vi "VoltageTest_R_VDC15V.vi"(0 "datain":string[](array[string])=["备注", "负载通道", "负载地址", "延时时间", "output max", "output min", "量测类型", "待测物板号"], 5 "HW CH Number":i32, 7 "Setup":string) -> (4 "REPORT INDECATE":string[][](array[string])=[["微安测试", "", "", "", ""], ["微安量测", "4", "0.000", "0.1", "NG"], ["微安量测", "4", "0.000", "0.1", "NG"], ["微安量测", "4", "0.000", "0.1", "NG"], ["微安量测", "4", "0.000", "0.1", "NG"]], 6 "ROW HEAD":string[](array[string]), 8 "PF":string[](array[string]), 10 "testData":string[](array[string]), 15 "Array":string[](array[string]))   [LabVIEW 2018]
uses:
  Subvi/Global.vi
panel:
  out "测试板数":i32
  out "数组":bool[](array[boolean])
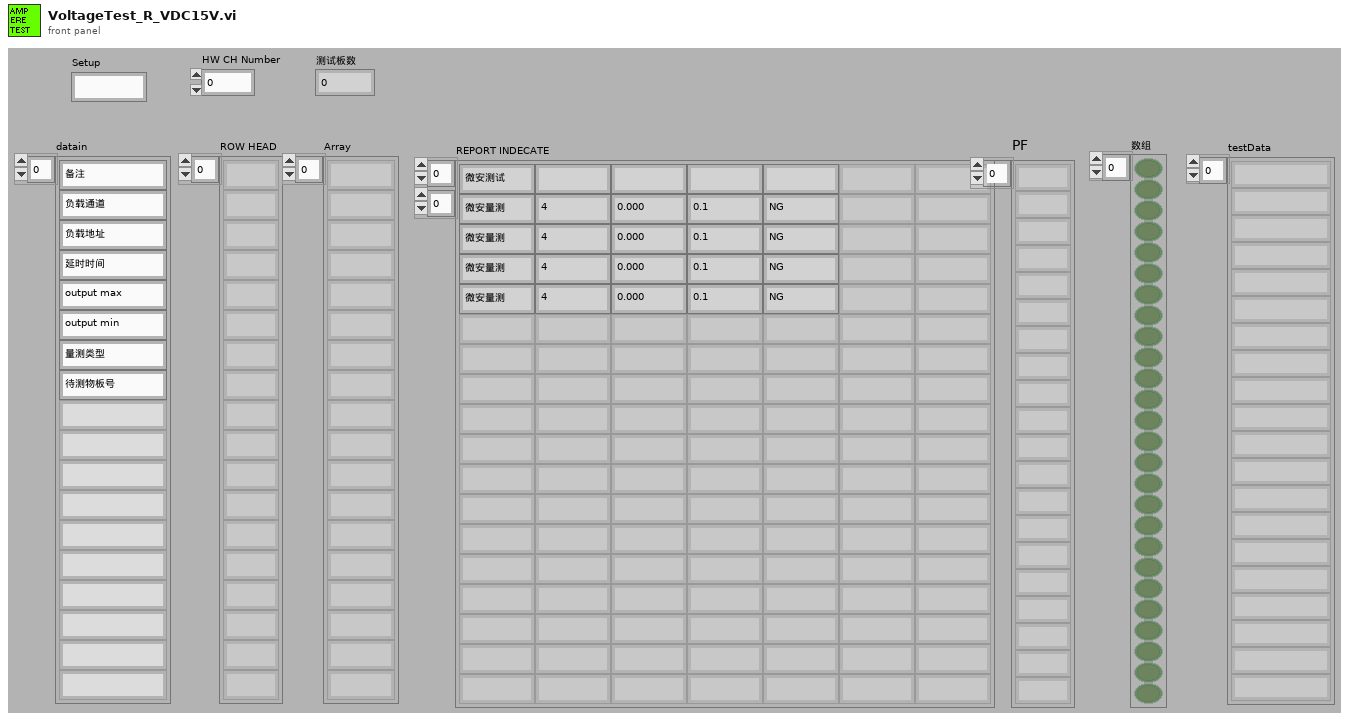
[diagram p1: front panel]
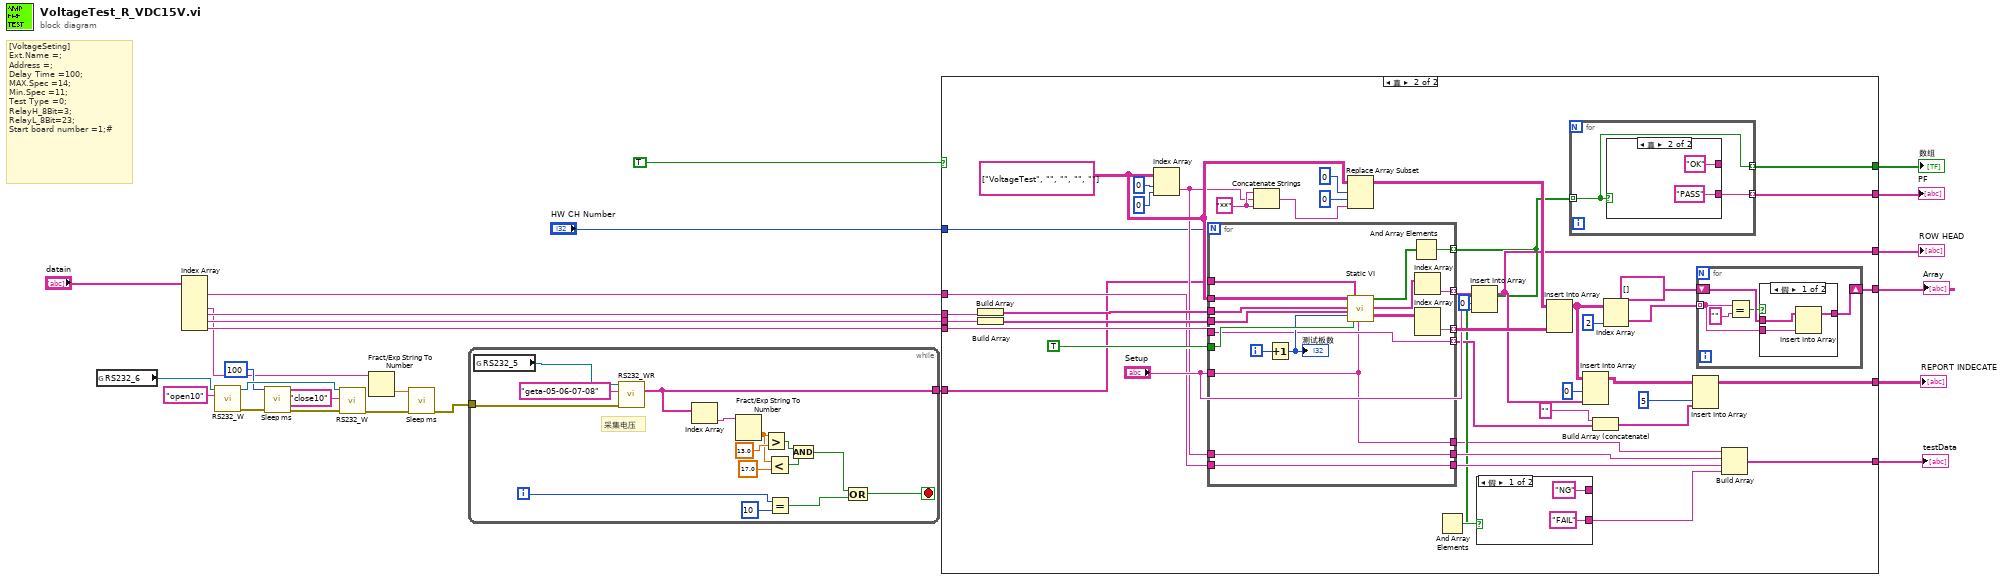
[diagram p0: block diagram]
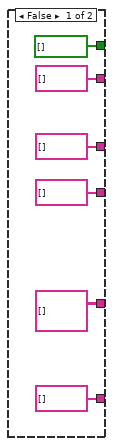
[diagram p2: hidden frame]
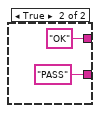
[diagram p3: hidden frame]
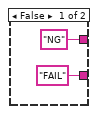
[diagram p4: hidden frame]
diagram:
  # "[VoltageSeting]\nExt.Name =;\nAddress =;\nDelay Time =100;\nMAX.Spec =14;\nMin.Spec =11;\nTest Type =0;\nRelayH_8Bit=3;\nRelayL_8Bit=23;\nStart board number =1;#"
  n1 = global read "Global.vi" "RS232_6"() -> (w11:refnum<visa-resource-name>)
  n2 = Index Array(array="datain") -> (element #1=w17:string, element #3=w2:string, element #4=w22:string, element #5=w21:string, element #6=w19:string)  [unwired: 6 in, 1 out]
  n3 = call "RS232_W.vi"("CMD"="open10", "VISA资源名称"=w11) -> ("error out"=w8:errorcluster, "VISA资源名称输出"=w10:refnum<visa-resource-name>)  [unwired: 7 in, 1 out]
  n4 = call "Sleep ms.vi"("error in (no error)"=w8, "等待时间（毫秒）"=u32 100) -> ("error out"=w9:errorcluster)  [unwired: 9 in]
  n5 = call "RS232_W.vi"("error in (no error)"=w9, "CMD"="close10", "VISA资源名称"=w10) -> ("error out"=w3:errorcluster)  [unwired: 6 in, 2 out]
  n6 = Fract/Exp String To Number(string=w2) -> (number=w4:dbl)  [unwired: 3 in, 1 out]
  n7 = call "Sleep ms.vi"("error in (no error)"=w3, "等待时间（毫秒）"=w4) -> ("error out"=w1:errorcluster)  [unwired: 9 in]
  n8 = while {
    tunnel: [w34] -> w13
    tunnel: w1 -> [w26]
    i -> [w33]
    stop <- w32 stop-if-true
    # "采集电压"
    n9 = global read "Global.vi" "RS232_5"() -> (w39:refnum<visa-resource-name>)
    n10 = call "RS232_WR.vi"("error in (no error)"=w26, "CMD"="geta-05-06-07-08", "VISA资源名称"=w39) -> ("Out data"=w34:string[])  [unwired: 6 in, 2 out]
    n11 = Index Array(array=w34) -> (element=w37:string)  [unwired: 1 in]
    n12 = Fract/Exp String To Number(string=w37) -> (number=w28:dbl)  [unwired: 3 in, 1 out]
    n13 = Greater?(x=w28, y=13.0) -> (0:w30:bool)
    n14 = Less?(x=w28, y=17.0) -> (x < y?=w31:bool)
    n15 = Equal?(x=w33, y=10) -> (x = y?=w38:bool)
    n16 = And(x=w30, y=w31) -> (x .and. y?=w29:bool)
    n17 = Compound Arithmetic op=OR ("复合运算")(w29, w38) -> (w32:bool)
  }
  n18 = case shown="真" TRUE {
    tunnel: [string[] [] ("Array") w87] -> w25
    tunnel: [string[] [] w86] -> w24
    tunnel: w22 -> [_ w79]
    tunnel: w21 -> [_ w78]
    tunnel: [string[] [] w67] -> w20
    tunnel: w19 -> [_ w65]
    tunnel: [string[][] [] w62] -> w18
    tunnel: w17 -> [_ w57]
    tunnel: [string[] [] w51] -> w16
    tunnel: [bool[] [] w49] -> w15
    tunnel: "HW CH Number" -> [_ w48]
    tunnel: w13 -> [_ w47]
    frame False {
    }
    frame True {
      w77 = string[][] [["VoltageTest", "", "", "", ""]]
      w83 = "**" ("字符串")
      n19 = Build Array(w79) -> (w76:string[])
      n20 = Build Array(w78) -> (w75:string[])
      n21 = Index Array(array=w77, index (row)=0 ("索引 (行)"), index (col)=0 ("禁用的索引 (列)")) -> (element=w58:string)
      n22 = for {
        N: w48 -> [_]
        tunnel: w47 -> [w111]
        tunnel: w76 -> [w109]
        tunnel: w75 -> [w108]
        tunnel: "Setup" -> [w95]
        tunnel: TRUE -> [w106]
        tunnel: [w104] -> w53 mode=indexing
        tunnel: [w101] -> w71 mode=indexing
        tunnel: w77 -> [w110]
        tunnel: [w99] -> w72 mode=indexing
        tunnel: w65 -> [w98]
        tunnel: [w98] -> w61 mode=indexing
        tunnel: w58 -> [w97]
        tunnel: [w97] -> w56
        tunnel: w57 -> [w96]
        tunnel: [w96] -> w55
        tunnel: [w95] -> w50
        i -> [w103]
        n23 = Increment(x=w103) -> (x+1=w105:i32)
        "测试板数" <- w105
        n24 = call "Static VI.vi"("添加的数组"=w110, "Max"=w109, "Min"=w108, "板数"=w105, "INPUTSTRING"=w111, "是否为字符串对比"=w106, "SQ"=w95) -> ("P/F"=w107:bool[], "SQ out"=w102:string[], "arrauy out"=w100:string[][])  [unwired: 9 in, 1 out]
        n25 = And Array Elements(Boolean array=w107) -> (logical AND=w104:bool)
        n26 = Index Array(array=w102) -> (element=w101:string)  [unwired: 1 in]
        n27 = Index Array(array=w100) -> (element=w99:string[])  [unwired: 2 in]
      }
      n28 = Concatenate Strings(w83, w58, w83) -> (w80:string)
      n29 = Replace Array Subset(array=w77, new element=w80, index (row)=0 ("索引 (行)"), index (col)=0 ("禁用的索引 (列)")) -> (w73:string[][])
      n30 = And Array Elements(Boolean array=w53) -> (logical AND=w54:bool)
      n31 = Insert Into Array(array=w71, index=0 ("索引"), new element="Setup") -> (w67:string[])
      n32 = case shown="假" w54 {
        tunnel: ["NG" "OK"] -> _
        tunnel: ["FAIL" "PASS"] -> w52
        frame False {
        }
        frame True {
        }
      }
      n33 = Insert Into Array ("数组插入")(array=w73, new element=w72) -> (w68:string[][])  [unwired: 2 in]
      n34 = for {
        tunnel: w53 -> [w112] mode=indexing
        tunnel: [w113] -> w86 mode=indexing
        tunnel: [w112] -> w49 mode=indexing
        n35 = case shown="真" w112 {
          tunnel: ["NG" "OK"] -> _
          tunnel: ["FAIL" "PASS"] -> w113
          frame False {
          }
          frame True {
          }
        }
      }
      n36 = Insert Into Array(array=w68, index (col)=0 ("禁用的索引 (列)"), new element=w67) -> (w63:string[][])  [unwired: 1 in]
      n37 = Build Array (concatenate)("" ("字符串"), w61) -> (w59:string[])
      n38 = Index Array(array=w68, index (col)=2 ("禁用的索引 (列)")) -> (element=w88:string[])  [unwired: 1 in]
      n39 = Insert Into Array(array=w63, index (col)=5 ("禁用的索引 (列)"), new element=w59) -> (w62:string[][])  [unwired: 1 in]
      n40 = for {
        tunnel: w88 -> [w118] mode=indexing
        shift-right: [w119] -> w87
        shift-left: string[] [] ("Array") -> [w122]
        n41 = Equal?(x=w118, y="") -> (x = y?=w120:bool)
        n42 = case shown="假" w120 {
          tunnel: w122 -> [w125 w126]
          tunnel: [w124 w126] -> w119
          tunnel: w118 -> [w123 _]
          frame False {
            n43 = Insert Into Array(array=w125, new element=w123) -> (w124:string[])  [unwired: 1 in]
          }
          frame True {
          }
        }
      }
      n44 = Build Array(w50, w56, w55, w52) -> (w51:string[])
    }
  }
  "REPORT INDECATE" <- w18
  "ROW HEAD" <- w20
  "PF" <- w24
  "Array" <- w25
  "数组" <- w15
  "testData" <- w16
